vi "Main.vi"() -> ()   [LabVIEW 2020]
uses:
  Connection Info.ctl
  Command.ctl
  Shared/MySQL/Preset Query Enum.ctl
  <userlib>/_OpenG.lib/array/array.llb/Index 1D Array Elements (String)__ogtk.vi
  <vilib>/Utility/tcp.llb/UDP Multicast Write-Only Open.vi
panel:
  in  "clear list":bool
  in  "Multicolumn Listbox":i32[](listbox)
  out "x+y":dbl
  in  "MultiCast Port":u16=58432
  in  "Multicast Address":string="234.5.6.7"
  in  "Multicast Local Port":u16=58431
  in  "Who Alive":bool
  out "Devies To Stop":string[](array[string])
  out "NewVal":i32[](array[numeric])
  out "All connections":T1[](array[typedef])
  in  "SendStop":bool
  in  "Exit":bool
  in  "Listbox":i32[](listbox)
  in  "error in (no error)":errorcluster
  out "Variant Out 2":variant
  out "Received String":string
  out "after substring 2":string
  out "Entity Name":string
  out "Entity IP address":string
  out "before substring 2":string
  out "before substring":string
  out "after substring":string
  out "data out":string
  in  "port":u16=6341
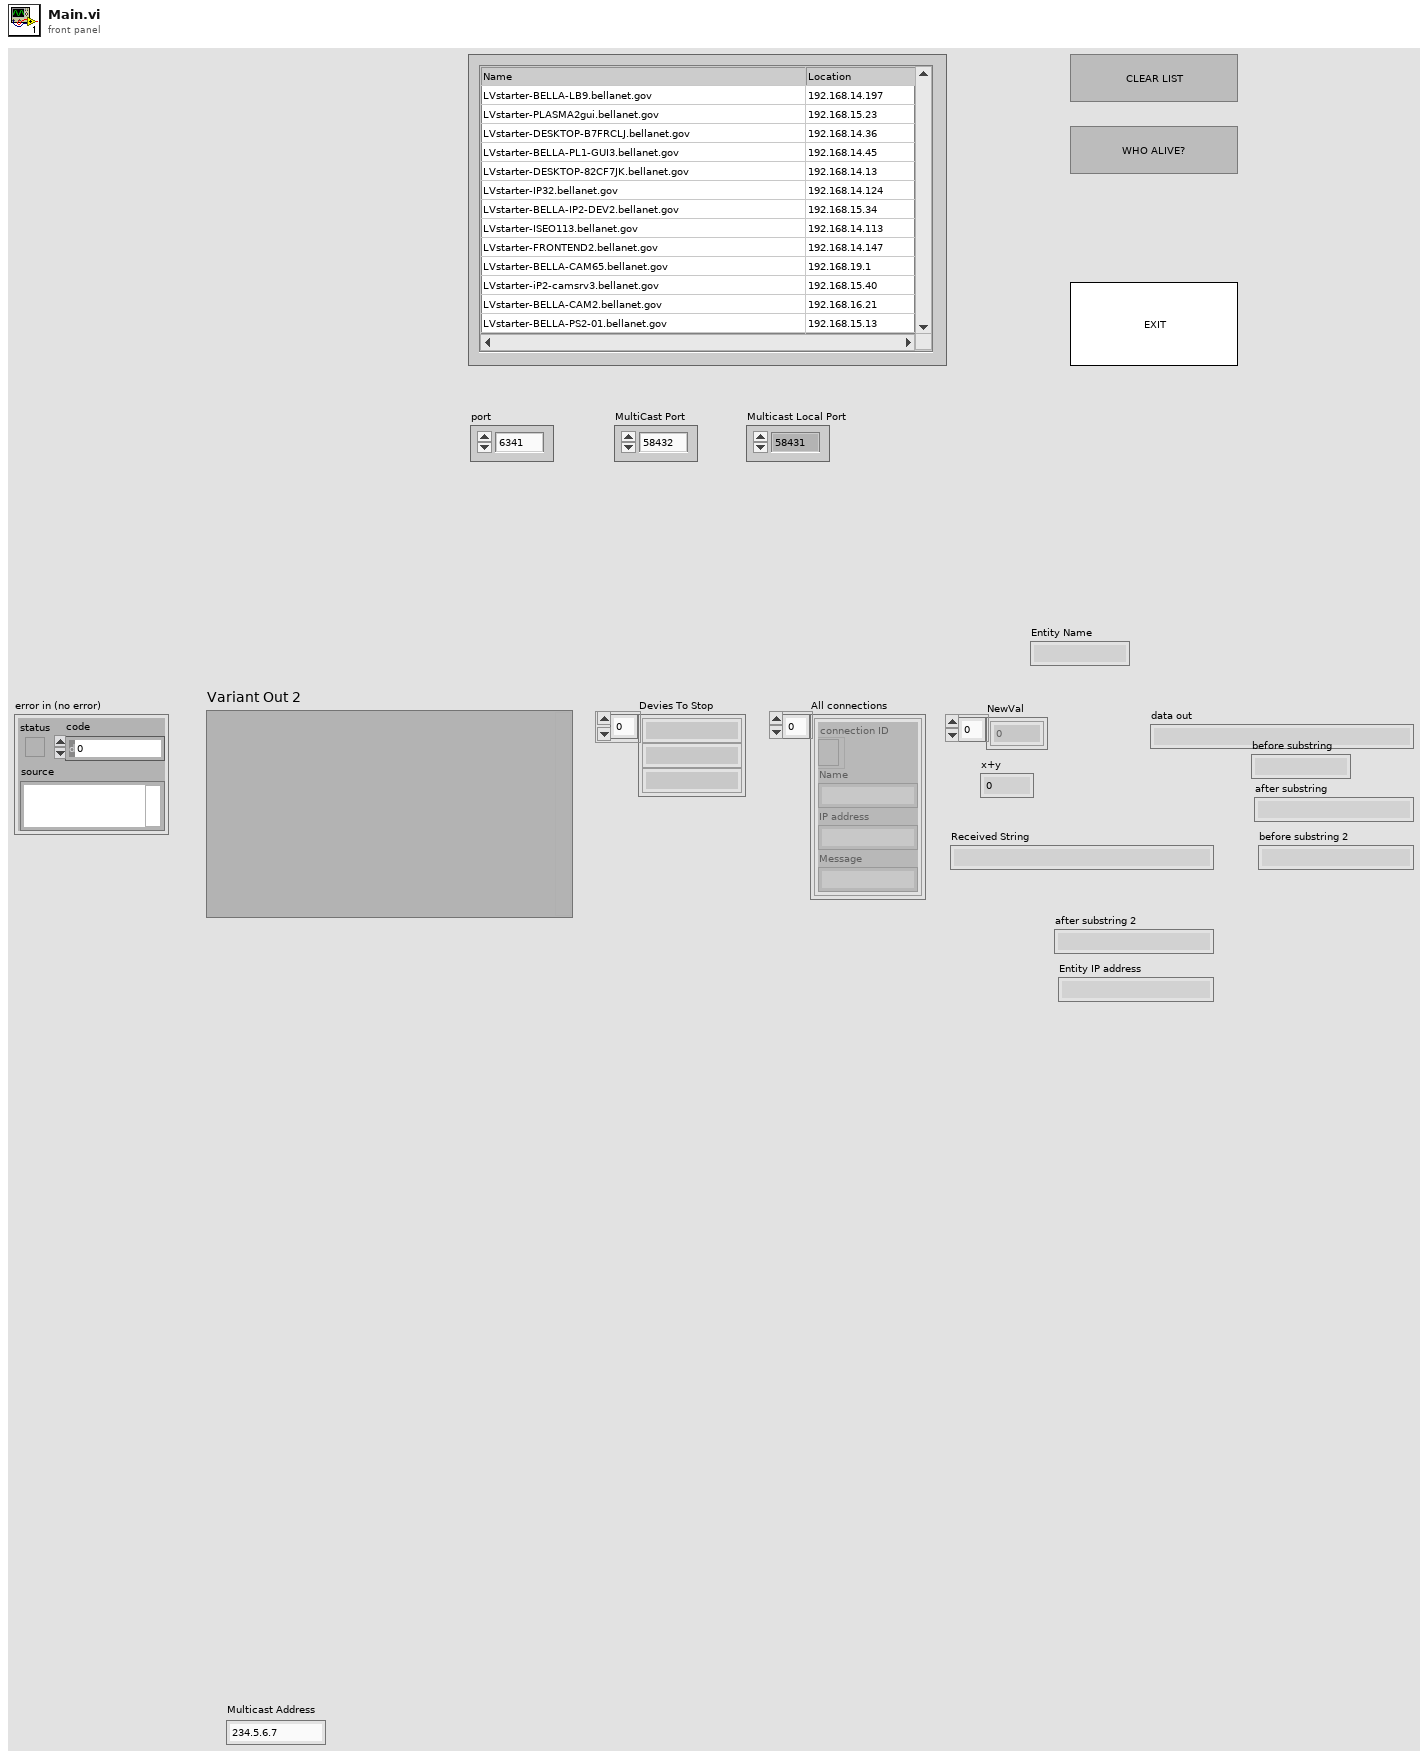
[diagram p1: front panel]
types:
  T1 = typedef "Connection Info.ctl" = cluster{"connection ID":refnum<k5>, "Name":string, "IP address":string, "Message":string}
  T2 = typedef "Command.ctl" = enum16{"add connection", "remove connection", "read connection data", "return all connections", "reset"}
  T3 = typedef "Preset Query Enum.ctl" = enum16{"Get Locations", "Get all IPs and MACs", "Get classes", "Get expt variables to set at scanstart for particular device", "Get expt devices and variables with start values", "Get expt devices and variables (with data to get)", "Get expt devices with data to get", "Get Expt devices and GUIs", "Get all devices basic properties", "Get Virtual Devices Core Info", "Get Expt names", "Get experiment basic properties", "Get experiment alarm variables", "Get MC Ports", "Get device network comm port", "Get devicetype lvclass path", "Get basic device properties", "Get Init Order", "Get all setable variables of a device", "Get device variable aliases", "Get force values of all settable variables", "Get all variables of a devicetype", "Get all variables of a device", "Get plotter details", "Get Saved Scans", "Get Scan Info", "GetGeneralGUIs", "Get expt for plotter", "Get plotter IDs from expt", "Get all devices", "Get all Virtual Devices", "Get all aliases", "Get variable and device info for Virtual Device", "GetItemLocatorIP", "Get IPs for GUIs", "Get DeviceType from Device", "GetLocalPortRange", "GetDevicePresetVariables", "Get Device Configuration", "GetAllPresetNames", "GetAllConfigurationNames", "GetPresetDeviceNames", "GetDeviceAliases", "GetDevicesOfClass"}
  T4 = enum32{"invalid app kind", "Development System", "Run Time System", "Student Edition", "Embedded LabVIEW", "Evaluation", "Custom"}
  T5 = enum32{"Invalid", "Standard", "Closed", "Hidden", "Minimized", "Maximized"}
  T6 = cluster{"Core":cluster{"Current VI Reference":refnum<vi>, "Close Panel on Exit?":bool}, "Your Boolean data":bool, "Your string data":string, "All connections":T1[], "Devies To Stop":string[], "MultiCast connection ID":refnum<k16>}
  T7 = cluster{"Current VI Reference":refnum<vi>, "Close Panel on Exit?":bool}
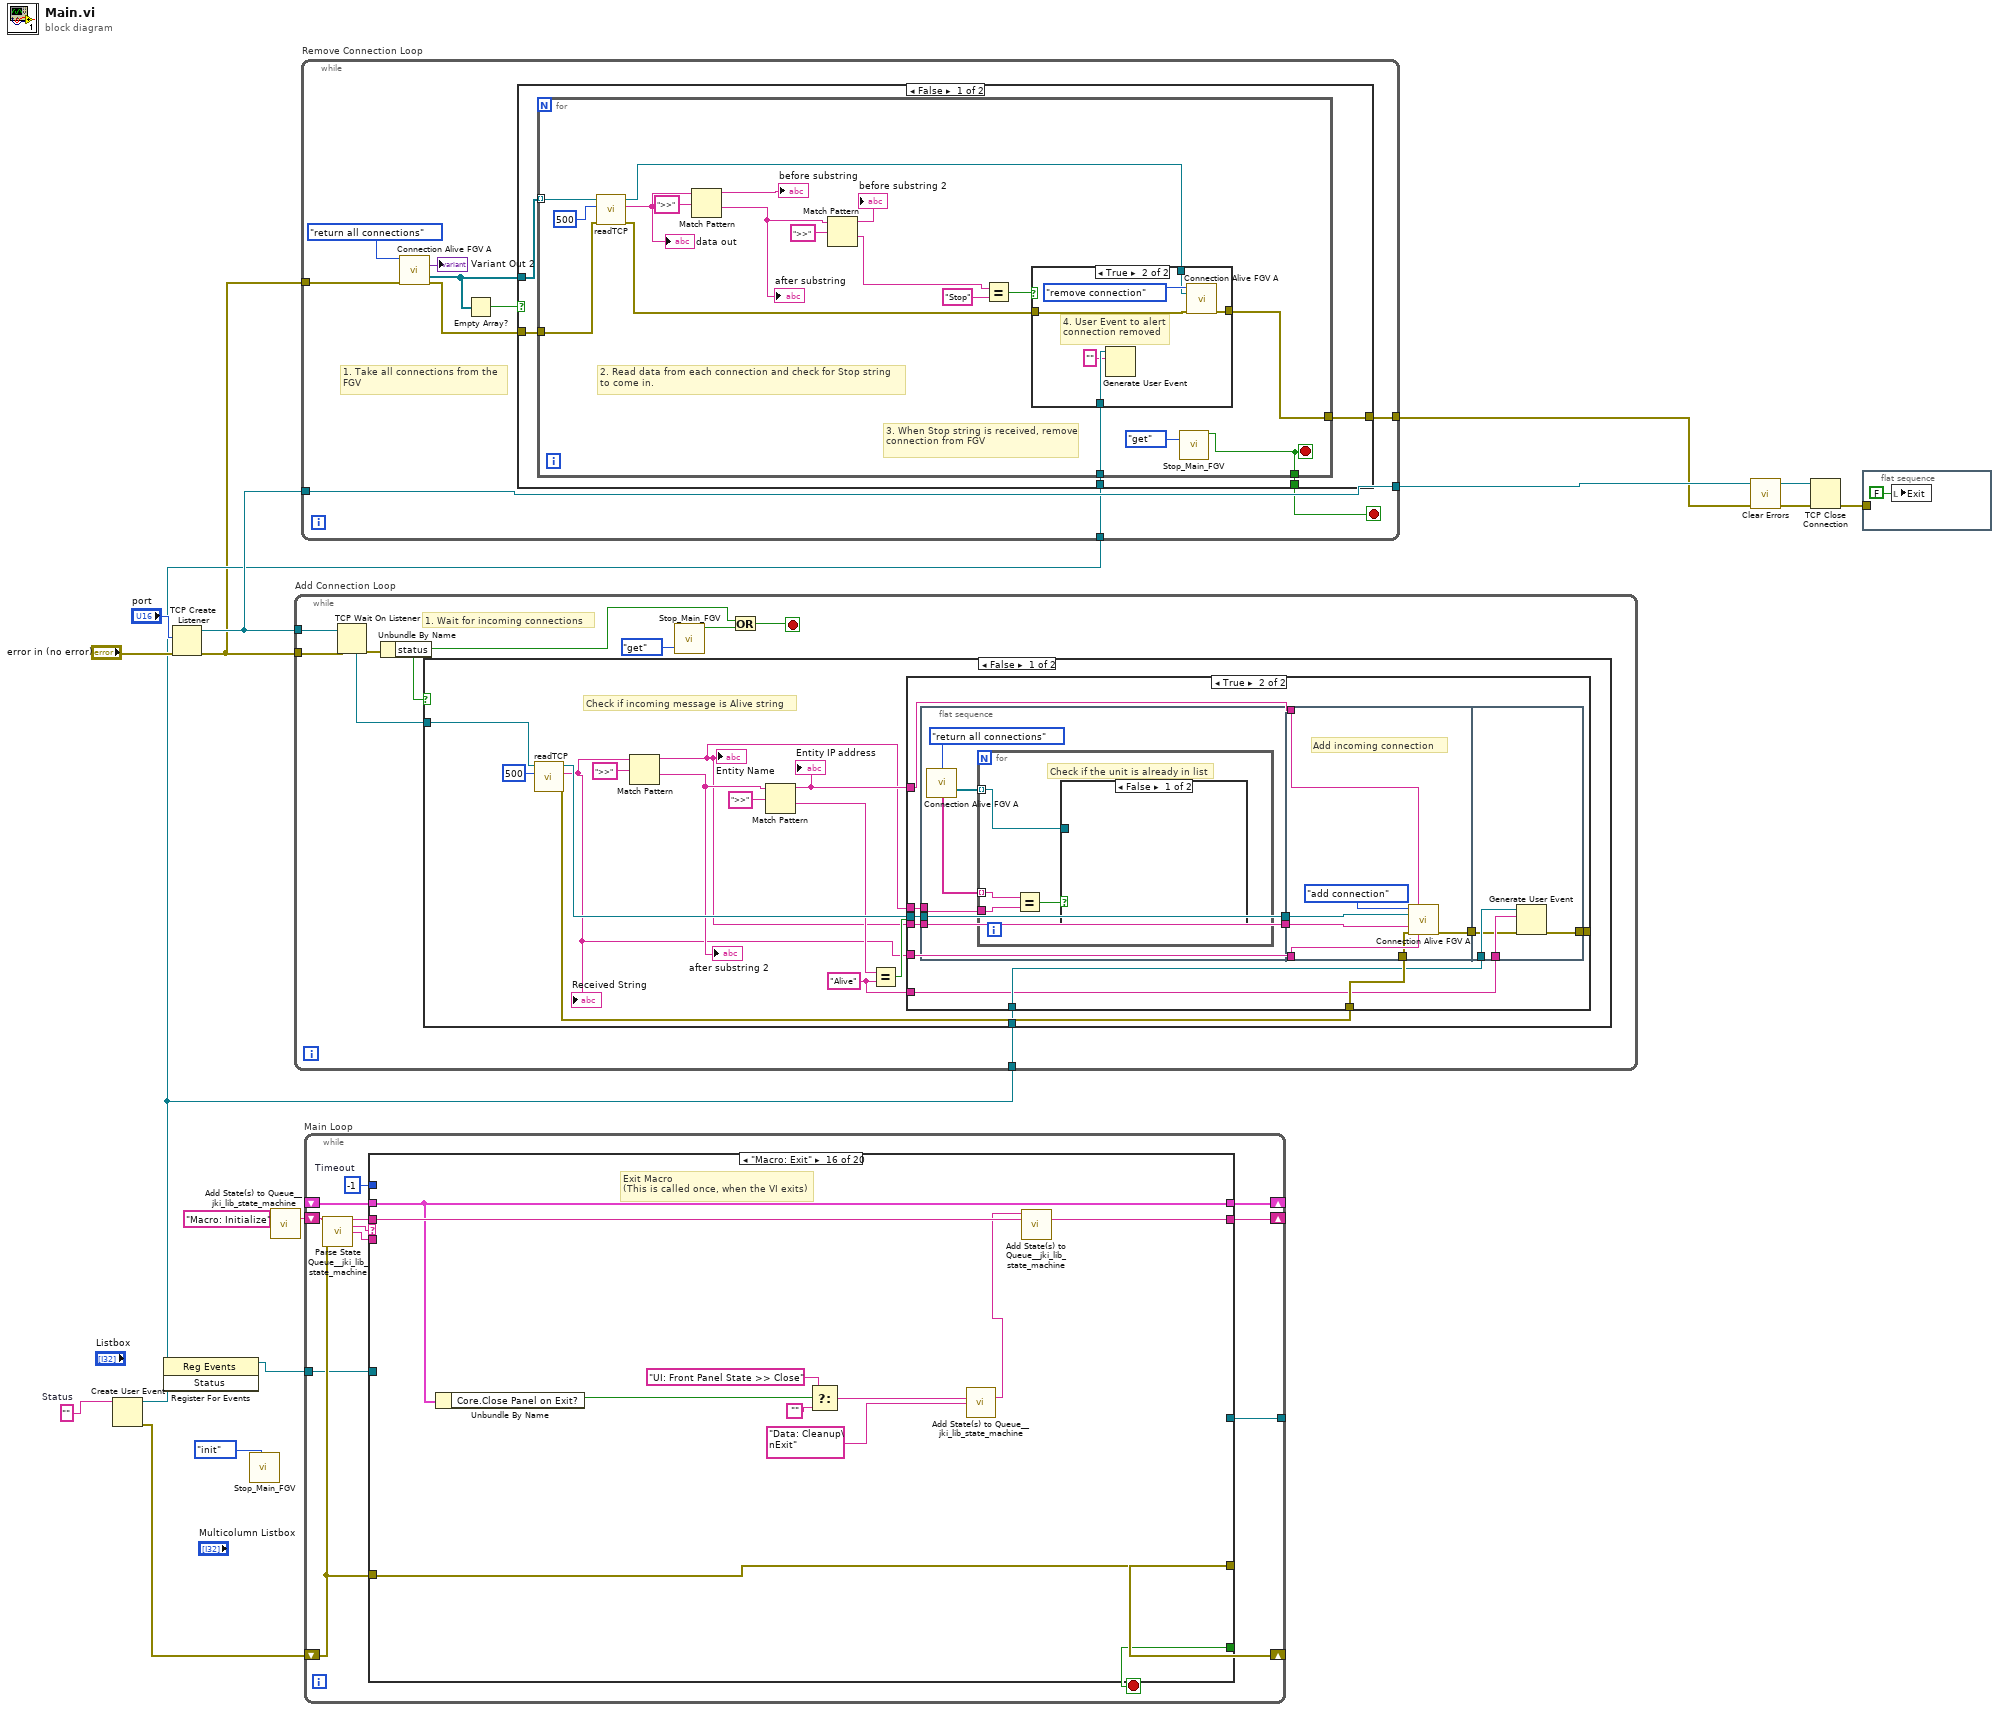
[diagram p0: block diagram]
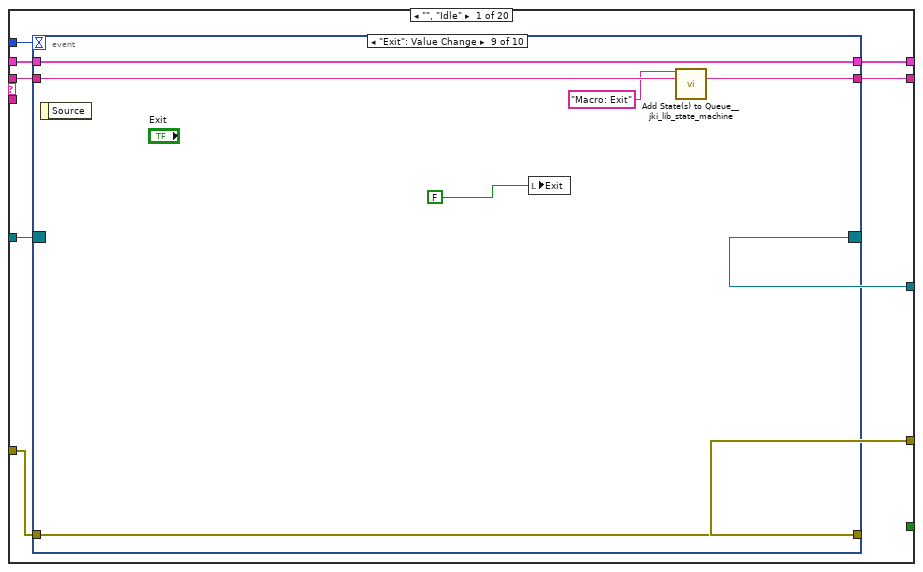
[diagram p2: hidden frame]
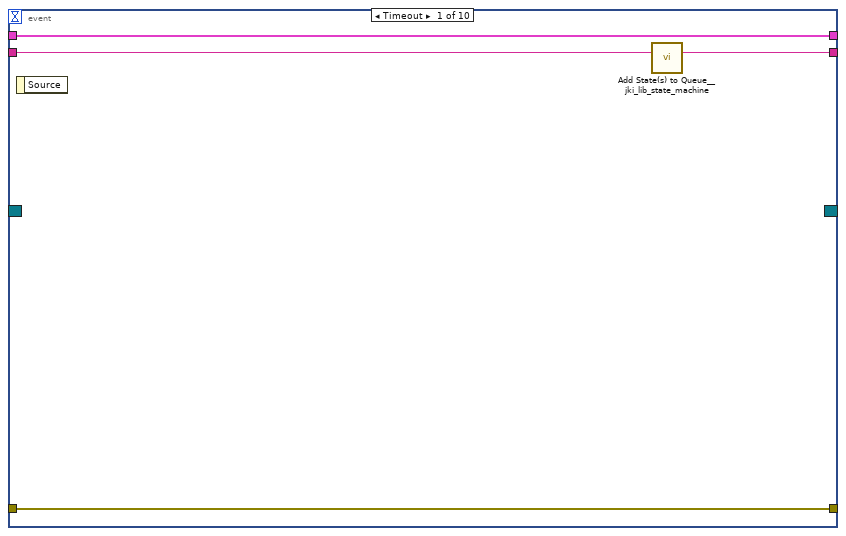
[diagram p3: hidden frame]
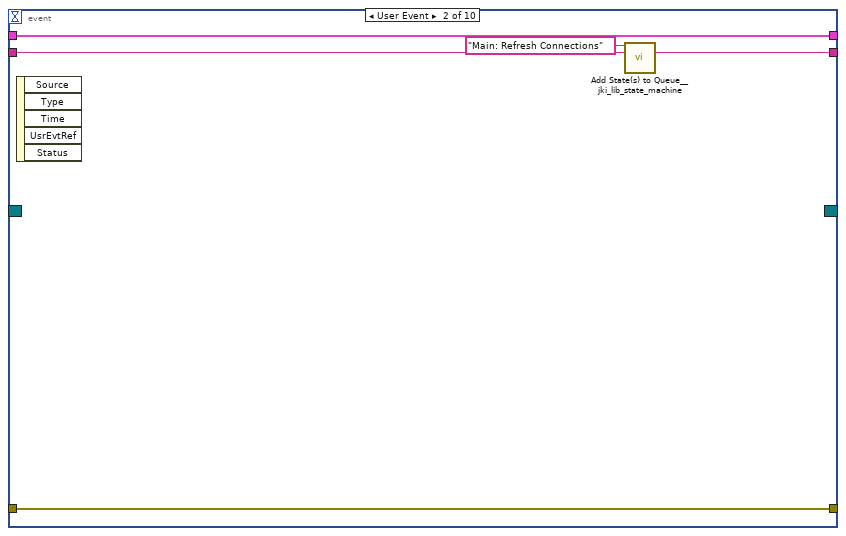
[diagram p4: hidden frame]
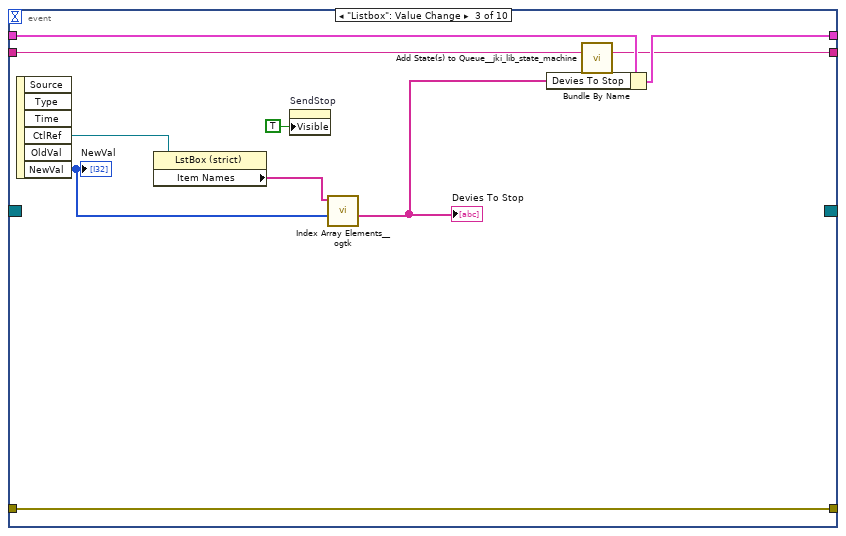
[diagram p5: hidden frame]
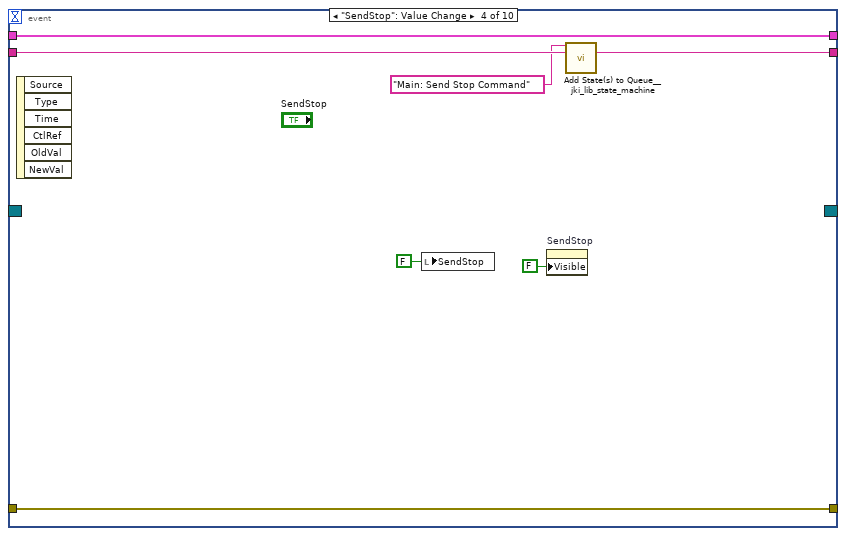
[diagram p6: hidden frame]
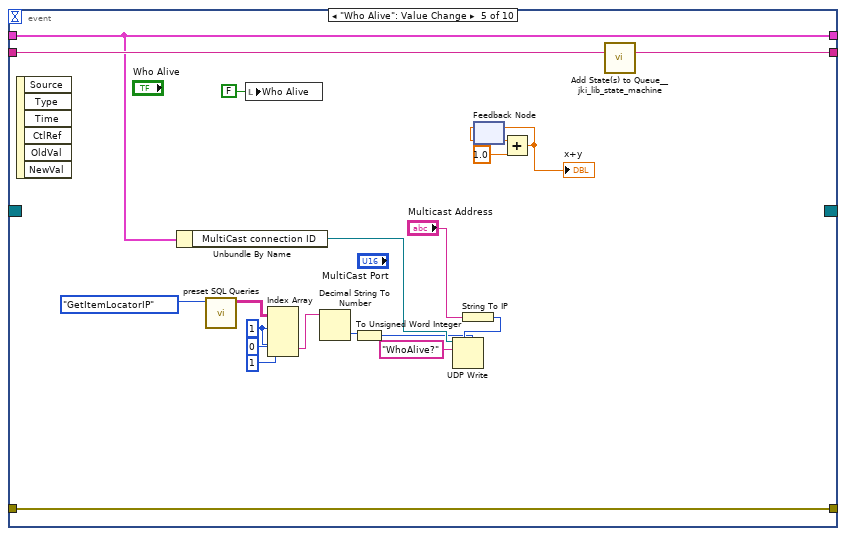
[diagram p7: hidden frame]
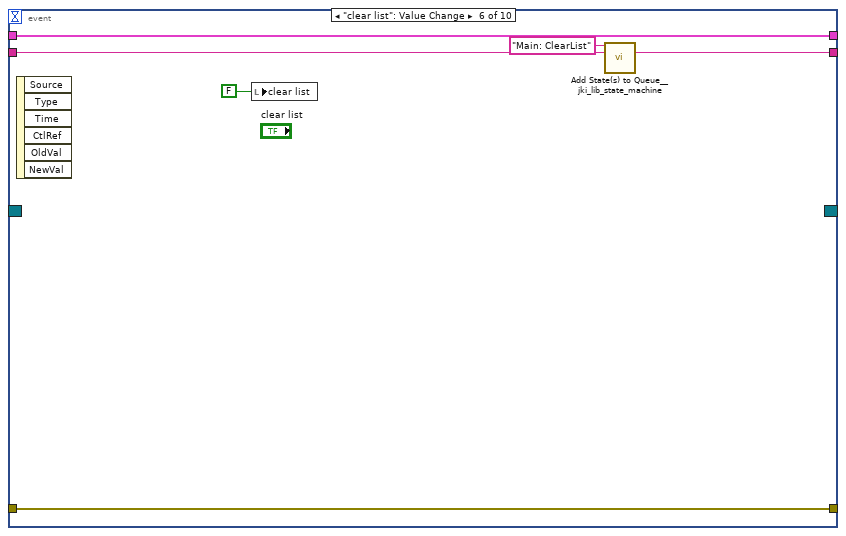
[diagram p8: hidden frame]
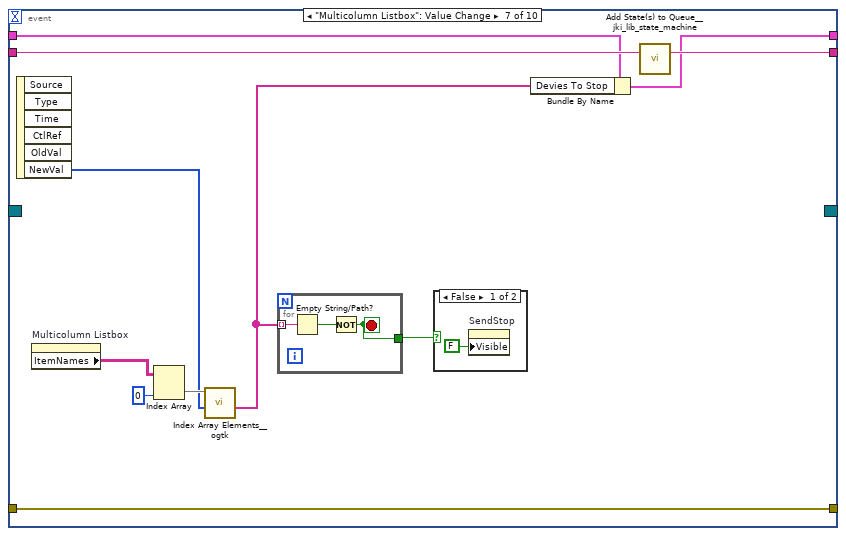
[diagram p9: hidden frame]
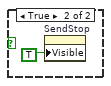
[diagram p10: hidden frame]
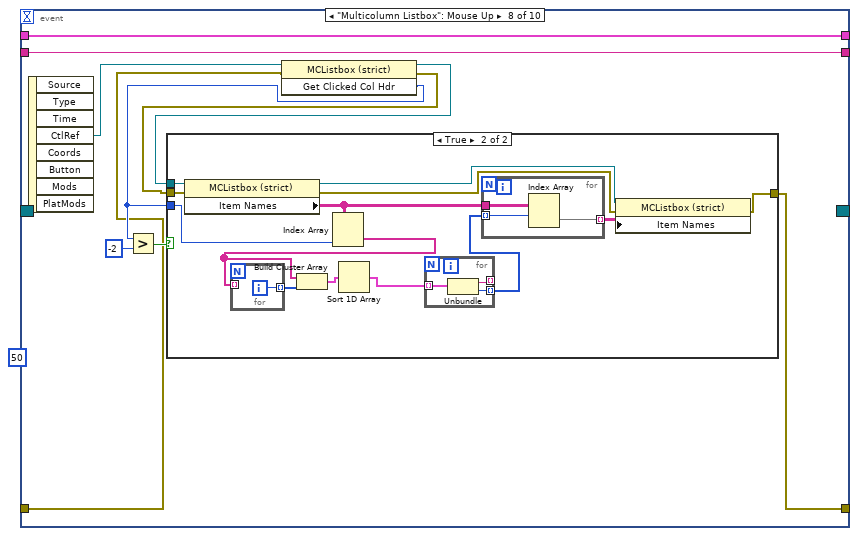
[diagram p11: hidden frame]
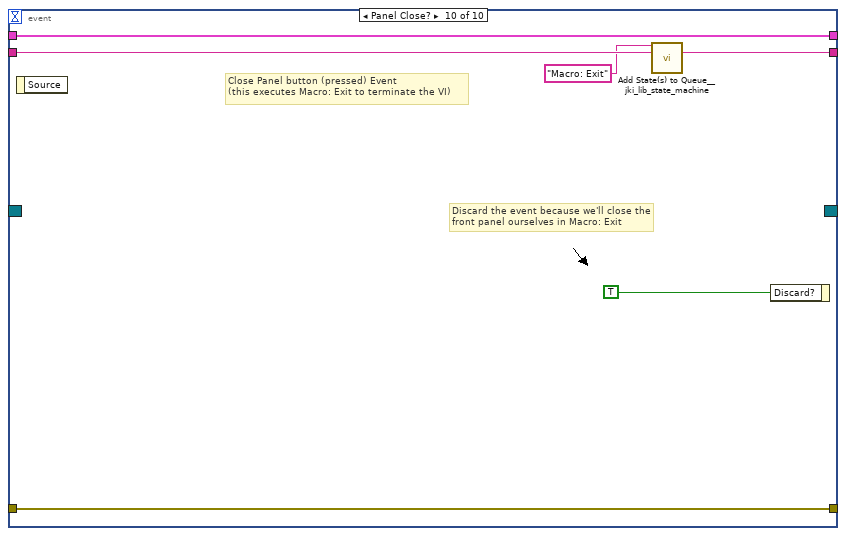
[diagram p13: hidden frame]
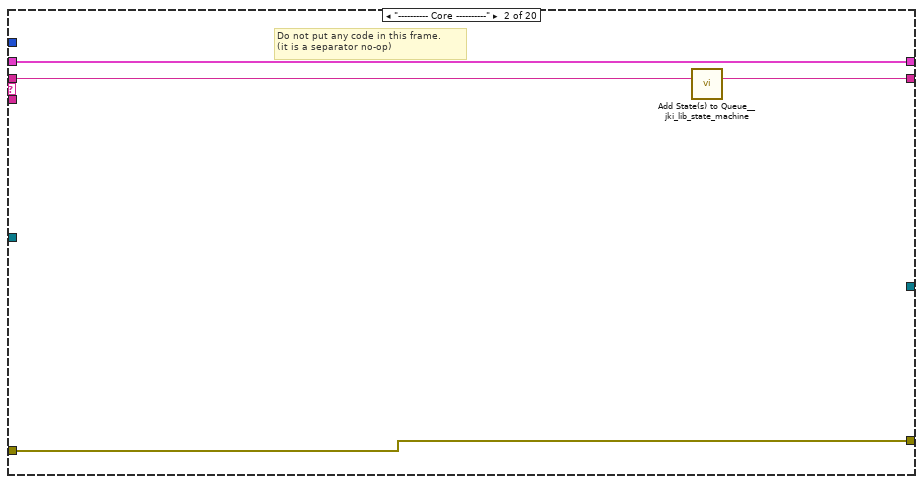
[diagram p14: hidden frame]
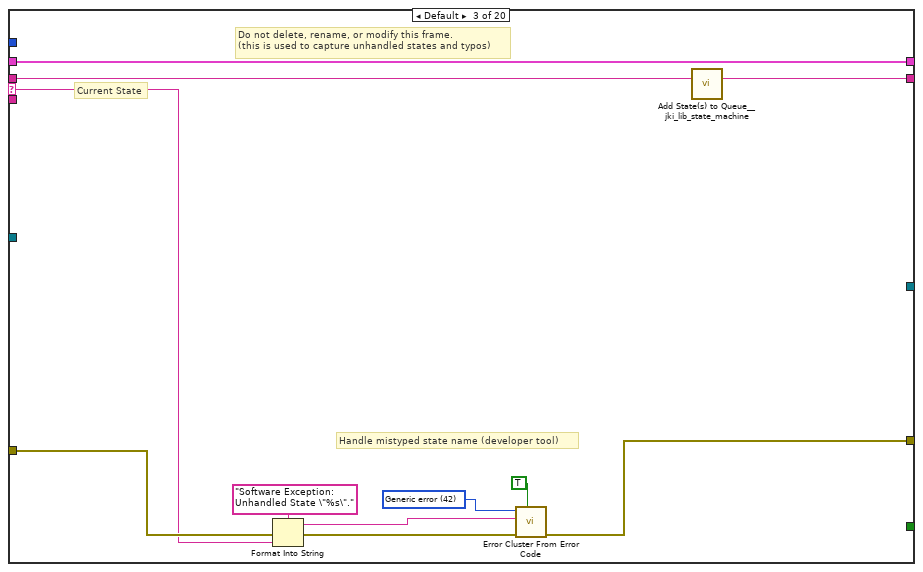
[diagram p15: hidden frame]
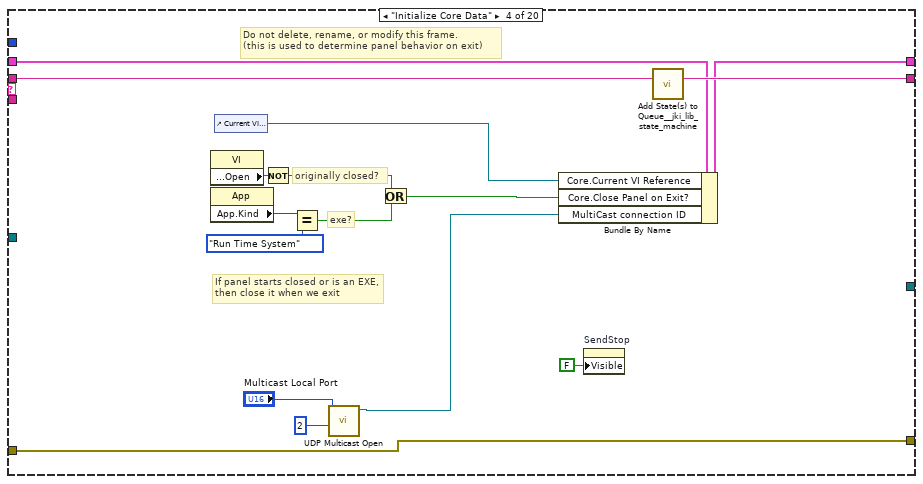
[diagram p16: hidden frame]
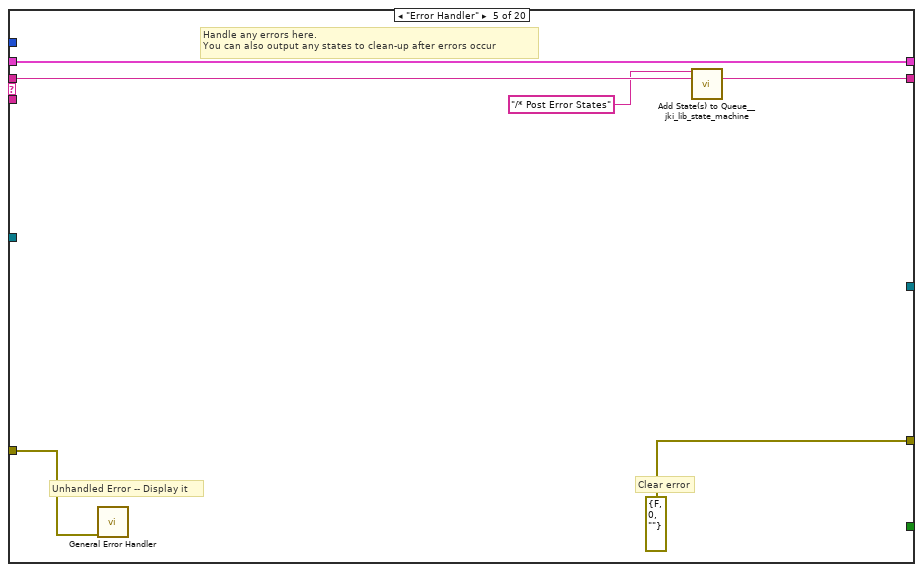
[diagram p17: hidden frame]
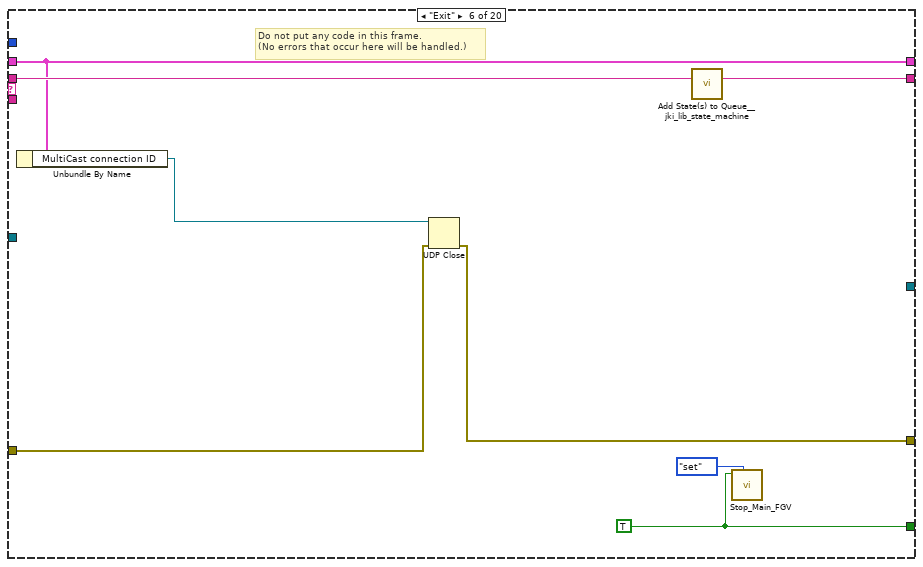
[diagram p18: hidden frame]
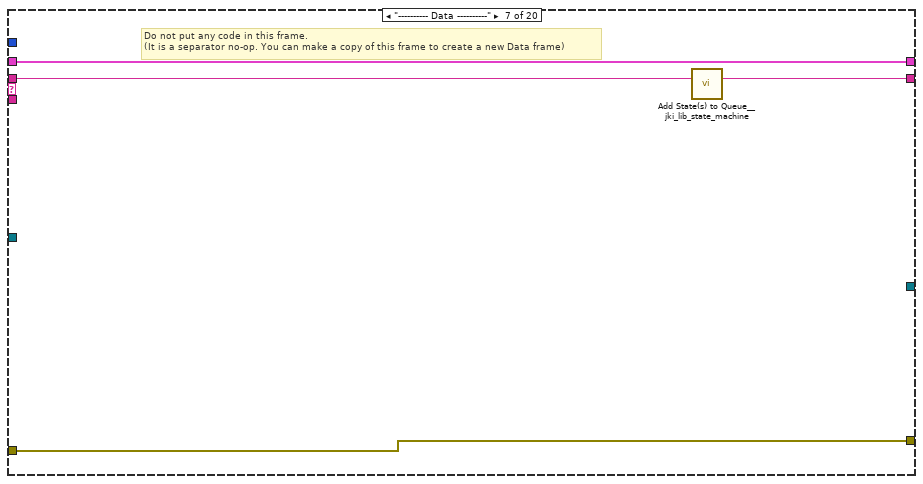
[diagram p19: hidden frame]
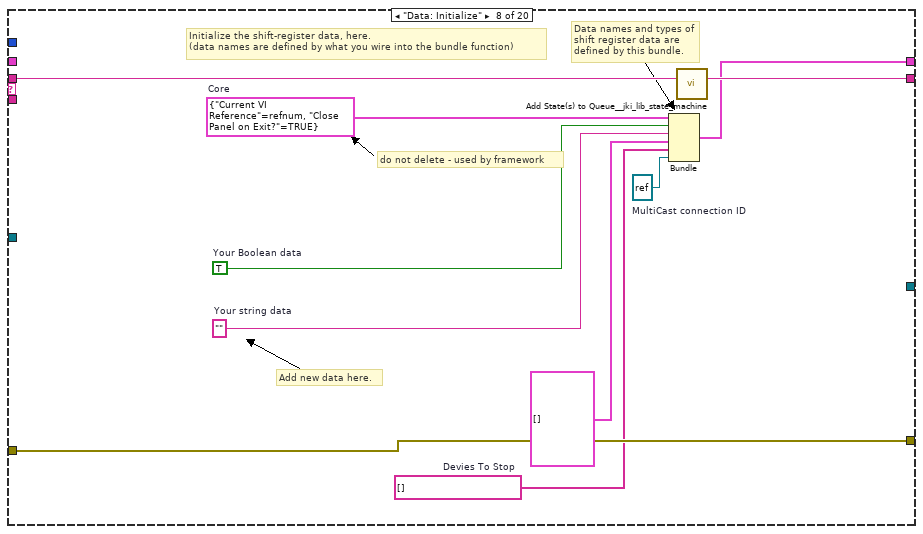
[diagram p20: hidden frame]
diagram:
  w6 = ""  # Status
  n1 = Create User Event(user event datatype=w6) -> (user event=w5:refnum<user-event>, error out=w3:errorcluster)  [unwired: 1 in]
  n2 = register-events(w5) -> (reference out=w7:refnum<event-registration>)  [unwired: 2 in, 1 out]
  n3 = TCP Create Listener(8:"error in (no error)", 10:"port") -> (0:w4:errorcluster, 3:w14:refnum<k5>)  [unwired: 4 out]
  n4 = call "Stop_Main_FGV.vi"("Command"=enum16{"set", "get", "init"}."init") -> ()  [unwired: 10 in, 1 out]
  n5 = call <vilib>:"Add State(s) to Queue__jki_lib_state_machine.vi"("State(s) in (\"\")"="Macro: Initialize") -> ("States Out"=w9:string)  [unwired: 14 in]
  n6 = while "Add Connection Loop" {
    tunnel: w4 -> [w24]
    tunnel: w14 -> [w23]
    tunnel: w5 -> [w20]
    stop <- w16 stop-if-true
    # "1. Wait for incoming connections"
    n7 = TCP Wait On Listener(8:w24, 11:w23) -> (0:w22:errorcluster, 4:w21:refnum<k5>)  [unwired: 5 out]
    n8 = Unbundle By Name(w22) -> ("status"=w17:bool)
    n9 = case shown="False" w17 {
      tunnel: w21 -> [w29 _]
      tunnel: w20 -> [w27 _]
      frame False {
        w26 = "Alive" ("y")
        # "Check if incoming message is Alive string"
        n10 = call "readTCP.vi"("timeout ms (-1)"=500, "connection ID in"=w29) -> ("error out"=w35:errorcluster, "data out"=w28:string, "connection ID out"=w37:refnum<k5>)  [unwired: 7 in]
        "Received String" <- w28
        n11 = Match Pattern(string=w28, regular expression=">>") -> (before substring=w25:string, after substring=w32:string)  [unwired: 1 in, 2 out]
        "after substring 2" <- w32
        "Entity Name" <- w25
        n12 = Match Pattern(string=w32, regular expression=">>") -> (before substring=w33:string, after substring=w36:string)  [unwired: 1 in, 2 out]
        "Entity IP address" <- w33
        n13 = Equal?(x=w36, y=w26) -> (x = y?=w34:bool)
        n14 = case shown="True" w34 {
          tunnel: w37 -> [_ w51]
          tunnel: w25 -> [_ w50]
          tunnel: w33 -> [_ w49]
          tunnel: [w39 w48] -> _
          tunnel: w28 -> [_ w47]
          tunnel: w35 -> [w39 w46]
          tunnel: w27 -> [_ w44]
          tunnel: w26 -> [_ w43]
          tunnel: w25 -> [_ w40]
          frame False {
          }
          frame True {
            n15 = flat-sequence {
              tunnel: w50 -> [w56]
              tunnel: w51 -> [w57]
              tunnel: [w57] -> w42
              tunnel: [w56] -> w41
              tunnel: w40 -> [w53]
              tunnel: w49 -> [w67]
              tunnel: w47 -> [w65]
              tunnel: w46 -> [w64]
              tunnel: [w66] -> w45
              tunnel: w42 -> [w70]
              tunnel: w41 -> [w68]
              tunnel: [w71] -> w48
              tunnel: w45 -> [w72]
              tunnel: w44 -> [w74]
              tunnel: w43 -> [w73]
              frame #0 {
                n16 = call "Connection Alive FGV A.vi"("command"=Command."return all connections") -> ("all connections"=w52:refnum<k5>[], "Names"=w54:string[])  [unwired: 7 in, 6 out]
                n17 = for {
                  tunnel: w54 -> [w61] mode=indexing
                  tunnel: w53 -> [w60]
                  tunnel: w52 -> [w58] mode=indexing
                  # "Check if the unit is already in list"
                  n18 = Equal?(x=w61, y=w60) -> (x = y?=w59:bool)
                  n19 = case shown="False" w59 {
                    tunnel: w58 -> [_ w62]
                    frame False {
                    }
                    frame True {
                      # "Remove existing connection"
                      n20 = call "Connection Alive FGV A.vi"("command"=Command."remove connection", "connection ID"=w62) -> ()  [unwired: 6 in, 8 out]
                    }
                  }
                }
              }
              frame #1 {
                # "Add incoming connection"
                n21 = call "Connection Alive FGV A.vi"("command"=Command."add connection", "IP address"=w67, "connection ID"=w70, "Name"=w68, "error in (no error)"=w64, "Message"=w65) -> ("error out"=w66:errorcluster)  [unwired: 2 in, 7 out]
              }
              frame #2 {
                n22 = Generate User Event(user event=w74, event data cluster=w73, error in=w72) -> (error out=w71:errorcluster)  [unwired: 1 in, 1 out]
              }
            }
          }
        }
      }
      frame True {
      }
    }
    n23 = call "Stop_Main_FGV.vi"("Command"=enum16{"set", "get", "init"}."get") -> ("Stop out"=w18:bool)  [unwired: 10 in]
    n24 = Or(x=w17, y=w18) -> (x .or. y?=w16:bool)
  }
  n25 = while "Remove Connection Loop" {
    tunnel: w14 -> [w80]
    tunnel: [w80] -> w13
    tunnel: [w79] -> w12
    tunnel: w5 -> [w77]
    tunnel: w4 -> [w76]
    stop <- w75 stop-if-true
    # "1. Take all connections from the \nFGV"
    n26 = call "Connection Alive FGV A.vi"("command"=Command."return all connections", "error in (no error)"=w76) -> ("Variant Out"=→"Variant Out 2":variant, "all connections"=w82:refnum<k5>[], "error out"=w83:errorcluster)  [unwired: 6 in, 5 out]
    n27 = Empty Array?(array=w82) -> (empty?=w81:bool)
    n28 = case shown="False" w81 {
      tunnel: w83 -> [w89 w117]
      tunnel: w82 -> [w88 _]
      tunnel: [w87 w117] -> w79
      tunnel: w77 -> [w86 _]
      tunnel: [w85 w115] -> w75
      frame False {
        n29 = for {
          tunnel: w88 -> [w107] mode=indexing
          tunnel: w89 -> [w96]
          tunnel: [w94] -> w87
          tunnel: w86 -> [w92]
          tunnel: [w90] -> w85
          stop <- w90 stop-if-true
          # "3. When Stop string is received, remove connection from FGV"
          # "2. Read data from each connection and check for Stop string\nto come in."
          n30 = call "readTCP.vi"("error in (no error)"=w96, "timeout ms (-1)"=500, "connection ID in"=w107) -> ("error out"=w95:errorcluster, "data out"=w93:string, "connection ID out"=w98:refnum<k5>)  [unwired: 6 in]
          "data out" <- w93
          n31 = Match Pattern(string=w93, regular expression=">>") -> (before substring=→"before substring":string, after substring=w103:string)  [unwired: 1 in, 2 out]
          "after substring" <- w103
          n32 = Match Pattern(string=w103, regular expression=">>") -> (before substring=→"before substring 2":string, after substring=w100:string)  [unwired: 1 in, 2 out]
          n33 = Equal?(x=w100, y="Stop") -> (x = y?=w99:bool)
          n34 = case shown="True" w99 {
            tunnel: w98 -> [_ w113]
            tunnel: [w108 w112] -> w94
            tunnel: w95 -> [w108 w111]
            tunnel: w92 -> [_ w110]
            frame False {
            }
            frame True {
              # "4. User Event to alert\nconnection removed"
              n35 = Generate User Event(user event=w110, event data cluster="" ("event data")) -> ()  [unwired: 2 in, 2 out]
              n36 = call "Connection Alive FGV A.vi"("command"=Command."remove connection", "connection ID"=w113, "error in (no error)"=w111) -> ("error out"=w112:errorcluster)  [unwired: 5 in, 7 out]
            }
          }
          n37 = call "Stop_Main_FGV.vi"("Command"=enum16{"set", "get", "init"}."get") -> ("Stop out"=w90:bool)  [unwired: 10 in]
        }
      }
      frame True {
        n38 = call "Stop_Main_FGV.vi"("Command"=enum16{"set", "get", "init"}."get") -> ("Stop out"=w115:bool)  [unwired: 10 in]
      }
    }
  }
  n39 = while "Main Loop" {
    shift-right: [w123] -> _
    shift-left: _ -> [w122]
    shift-right: [w126] -> _
    shift-left: w3 -> [w120]
    shift-right: [w125] -> _
    shift-left: w9 -> [w127]
    tunnel: w7 -> [w119]
    tunnel: [w118] -> _
    stop <- w124 stop-if-true
    w121 = -1  # Timeout
    n40 = call <vilib>:"Parse State Queue__jki_lib_state_machine.vi"("State Queue"=w127, "Error In (no error)"=w120) -> ("Remaining States"=w129:string, "Current State"=w130:string, "Arguments"=w128:string)  [unwired: 11 in]
    n41 = case shown="\"Macro: Exit\"" w130 {
      selector: w130 -> [_ _ w255 _ _ _ _ _ _ _ _ _ _ _ _ _ _ _ _ _]
      tunnel: w129 -> [w139 w254 w259 w281 w287 w295 w299 w309 w315 w319 w323 w329 w340 w366 w371 w381 w385 w391 w417 w432]
      tunnel: w128 -> [_ _ _ _ _ _ _ _ _ _ _ w324 w334 _ _ _ _ _ _ _]
      tunnel: w122 -> [w137 w251 w257 w272 w284 w293 w296 _ w310 w316 w321 w327 w336 w363 w368 w378 w382 w388 w414 w421]
      tunnel: [w136 w252 w261 w278 errorcluster {"status"=FALSE, "code"=0, "source"=""} ("error out") w290 w297 w306 w311 w317 w320 w325 w337 w364 w369 w379 w383 w389 w415 w430] -> w126
      tunnel: w120 -> [w135 w252 w260 w278 w283 w291 w297 w306 w312 w317 w320 w326 w338 w364 w369 w379 w383 w389 w415 w430]
      tunnel: [w138 w253 w258 w280 w286 w294 w298 w308 w314 w318 w322 w328 w339 w365 w370 w380 w384 w390 w416 w431] -> w125
      tunnel: [_ _ _ _ _ w289 _ _ _ _ _ _ _ _ _ _ _ _ _ _] -> w124
      tunnel: [w134 w251 w257 w279 w284 w293 w296 w307 w310 w316 w321 w327 w336 w363 w368 w378 w382 w388 w414 w420] -> w123
      tunnel: w121 -> [w133 _ _ _ _ _ _ _ _ _ _ _ _ _ _ _ _ _ _ _]
      tunnel: w119 -> [w132 _ _ _ _ _ _ _ _ _ _ _ _ _ _ _ _ _ _ _]
      tunnel: [w131 _ _ _ _ _ _ _ _ _ _ _ _ _ _ _ _ _ _ _] -> w118
      frame "", "Idle" {
        n42 = event shown="[8] \"Exit\": Value Change" {
          selector: w132 -> [_ _ _ _ _ _ _ _ _ _]
          dyn-events: [_ _ _ _ _ _ _ _ _ _] -> w131
          timeout: w133 -> [_ _ _ _ _ _ _ _ _ _]
          tunnel: w139 -> [w143 w146 w150 w163 w179 w188 w201 w208 w244 w250]
          tunnel: [w142 w147 w149 w162 w180 w189 w202 w208 w243 w249] -> w138
          tunnel: w137 -> [w140 w144 w153 w165 w178 w187 w195 w209 w241 w247]
          tunnel: [w141 w148 w157 w164 w181 w190 w198 w210 w242 w248] -> w136
          tunnel: w135 -> [w141 w148 w157 w164 w181 w190 w198 w213 w242 w248]
          tunnel: [w140 w144 w152 w165 w178 w187 w194 w209 w241 w247] -> w134
          event Timeout {
            n43 = event-data() -> ()  [unwired: 1 in, 1 out]
            n44 = call <vilib>:"Add State(s) to Queue__jki_lib_state_machine.vi"("State(s) in (\"\")"=w143) -> ("States Out"=w142:string)  [unwired: 14 in]
          }
          event User Event {
            n45 = event-data() -> ()  [unwired: 1 in, 5 out]
            n46 = call <vilib>:"Add State(s) to Queue__jki_lib_state_machine.vi"("State(s) in Front (\"\")"="Main: Refresh Connections" ("State(s) in Front (\"\")"), "State(s) in (\"\")"=w146) -> ("States Out"=w147:string)  [unwired: 13 in]
          }
          event "Listbox": Value Change {
            n47 = event-data() -> ("CtlRef"=w156:refnum<vi>, "NewVal"=w154:i32[])  [unwired: 1 in, 4 out]
            "NewVal" <- w154
            n48 = property class="LstBox (strict)"(reference=w156) -> ("Item Names"=w155:string[])  [unwired: 1 in, 2 out]
            n49 = property on="SendStop" class="Bool (strict)"("Visible"=TRUE) -> ()  [unwired: 2 in, 2 out]
            n50 = call-poly <userlib>:"Index Array Elements__ogtk.vi"("indices"=w154, "array"=w155) -> ("elements"=w151:string[])  [unwired: 9 in]
            "Devies To Stop" <- w151
            n51 = Bundle By Name(cluster=w153, "Devies To Stop"=w151) -> (w152:T6)
            n52 = call <vilib>:"Add State(s) to Queue__jki_lib_state_machine.vi"("State(s) in (\"\")"=w150) -> ("States Out"=w149:string)  [unwired: 14 in]
          }
          event "SendStop": Value Change {
            n53 = event-data() -> ()  [unwired: 1 in, 6 out]
            n54 = local write "SendStop"(FALSE ("OK 2")) -> ()
            n55 = property on="SendStop" class="Bool (strict)"("Visible"=FALSE) -> ()  [unwired: 2 in, 2 out]
            n56 = call <vilib>:"Add State(s) to Queue__jki_lib_state_machine.vi"("State(s) in Front (\"\")"="Main: Send Stop Command" ("State(s) in Front (\"\")"), "State(s) in (\"\")"=w163) -> ("States Out"=w162:string)  [unwired: 13 in]
          }
          event "Who Alive": Value Change {
            w168 = 1 ("index (row)")
            n57 = event-data() -> ()  [unwired: 1 in, 6 out]
            n58 = Unbundle By Name(w178) -> ("MultiCast connection ID"=w177:refnum<k16>)
            n59 = call "preset SQL Queries.vi"("Preset Query"=Preset_Query_Enum."GetItemLocatorIP") -> ("data"=w167:string[][])  [unwired: 8 in, 2 out]
            n60 = local write "Who Alive"(FALSE ("Who Alive")) -> ()
            n61 = Index Array(array=w167, index (row) #1=w168, index (col) #1=0 ("disabled index (col)"), index (row) #2=w168, index (col) #2=1 ("disabled index (col)")) -> (element #2=w166:string)  [unwired: 1 out]
            n62 = Decimal String To Number(string=w166) -> (number=w172:i32)  [unwired: 2 in, 1 out]
            n63 = To Unsigned Word Integer(number=w172) -> (unsigned 16bit integer=w171:u16)
            n64 = String To IP(1:"Multicast Address") -> (0:w183:u32)
            n65 = UDP Write(address=w183, port or service name=w171, connection ID=w177, data in="WhoAlive?") -> ()  [unwired: 2 in, 2 out]
            n66 = feedback #1() -> (w175:dbl)  [unwired: 1 in]
            n67 = Add(x=w175, y=1.0) -> (x+y=w176:dbl)
            "x+y" <- w176
            n68 = feedback-in #1(w176) -> ()
            n69 = call <vilib>:"Add State(s) to Queue__jki_lib_state_machine.vi"("State(s) in (\"\")"=w179) -> ("States Out"=w180:string)  [unwired: 14 in]
          }
          event "clear list": Value Change {
            n70 = event-data() -> ()  [unwired: 1 in, 6 out]
            n71 = local write "clear list"(FALSE ("Who Alive")) -> ()
            n72 = call <vilib>:"Add State(s) to Queue__jki_lib_state_machine.vi"("State(s) in Front (\"\")"="Main: ClearList" ("State(s) in Front (\"\")"), "State(s) in (\"\")"=w188) -> ("States Out"=w189:string)  [unwired: 13 in]
          }
          event "Multicolumn Listbox": Value Change {
            n73 = event-data() -> ("NewVal"=w196:i32[])  [unwired: 1 in, 5 out]
            n74 = property on="Multicolumn Listbox" class="MCListbox (strict)"() -> ("ItemNames"=w200:string[][])  [unwired: 2 in, 2 out]
            n75 = Index Array(array=w200, index (col)=0 ("disabled index (col)")) -> (element=w197:string[])  [unwired: 1 in]
            n76 = call-poly <userlib>:"Index Array Elements__ogtk.vi"("indices"=w196, "array"=w197) -> ("elements"=w193:string[])  [unwired: 9 in]
            n77 = for {
              tunnel: w193 -> [w207] mode=indexing
              tunnel: [w205] -> w192
              stop <- w205 stop-if-true
              n78 = Empty String/Path?(string/path=w207) -> (empty?=w206:bool)
              n79 = Not(x=w206) -> (.not. x?=w205:bool)
            }
            n80 = case shown="False" w192 {
              frame False {
                n81 = property on="SendStop" class="Bool (strict)"("Visible"=FALSE) -> ()  [unwired: 2 in, 2 out]
              }
              frame True {
                n82 = property on="SendStop" class="Bool (strict)"("Visible"=TRUE) -> ()  [unwired: 2 in, 2 out]
              }
            }
            n83 = Bundle By Name(cluster=w195, "Devies To Stop"=w193) -> (w194:T6)
            n84 = call <vilib>:"Add State(s) to Queue__jki_lib_state_machine.vi"("State(s) in (\"\")"=w201) -> ("States Out"=w202:string)  [unwired: 14 in]
          }
          event "Multicolumn Listbox": Mouse Up {
            (unwired) u32 50 ("milliseconds to wait")
            n85 = event-data() -> ("CtlRef"=w215:refnum<vi>)  [unwired: 1 in, 7 out]
            n86 = invoke class="MCListbox (strict)" method="Get Clicked Col Hdr"(reference=w215, error in=w213) -> (reference out=w212:refnum<vi>, error out=w211:errorcluster, "Get Clicked Column Header"=w214:i32)  [unwired: 1 in]
            n87 = Greater?(x=w214, y=-2) -> (0:w217:bool)
            n88 = case shown="True" w217 {
              tunnel: w214 -> [_ w231]
              tunnel: w211 -> [w218 w224]
              tunnel: w212 -> [_ w230]
              tunnel: [w218 w225] -> w210
              frame False {
              }
              frame True {
                n89 = property class="MCListbox (strict)"(reference=w230, error in=w224) -> (reference out=w226:refnum<vi>, error out=w227:errorcluster, "Item Names"=w229:string[][])
                n90 = Index Array(array=w229, index (col)=w231) -> (element=w220:string[])  [unwired: 1 in]
                n91 = for {
                  tunnel: [w235] -> w221 mode=indexing
                  tunnel: w220 -> [_] mode=indexing
                  i -> [w235]
                }
                n92 = Build Cluster Array ("Index & Bundle Cluster Array")(w220, w221) -> (w222:cluster{string, i32}[])
                n93 = Sort 1D Array(array=w222) -> (sorted array=w223:cluster{string, i32}[])
                n94 = for {
                  tunnel: w223 -> [w234] mode=indexing
                  tunnel: [w233] -> _ mode=indexing
                  tunnel: [w232] -> w219 mode=indexing
                  n95 = Unbundle(w234) -> (w233:string, w232:i32)
                }
                n96 = for {
                  tunnel: w219 -> [w237] mode=indexing
                  tunnel: w229 -> [w238]
                  tunnel: [w236] -> w228 mode=indexing
                  n97 = Index Array(array=w238, index (row)=w237) -> (element=w236:string[])  [unwired: 1 in]
                }
                n98 = property class="MCListbox (strict)"(reference=w226, error in=w227, "Item Names"=w228) -> (error out=w225:errorcluster)  [unwired: 1 out]
              }
            }
          }
          event "Exit": Value Change {
            n99 = event-data() -> ()  [unwired: 1 in, 1 out]
            n100 = local write "Exit"(FALSE ("OK")) -> ()
            n101 = call <vilib>:"Add State(s) to Queue__jki_lib_state_machine.vi"("State(s) in Front (\"\")"="Macro: Exit", "State(s) in (\"\")"=w244) -> ("States Out"=w243:string)  [unwired: 13 in]
          }
          event Panel Close? {
            # "Discard the event because we'll close the front panel ourselves in Macro: Exit"
            # "Close Panel button (pressed) Event\n(this executes Macro: Exit to terminate the VI)"
            n102 = event-data() -> ()  [unwired: 1 in, 1 out]
            n103 = call <vilib>:"Add State(s) to Queue__jki_lib_state_machine.vi"("State(s) in Front (\"\")"="Macro: Exit", "State(s) in (\"\")"=w250) -> ("States Out"=w249:string)  [unwired: 13 in]
            n104 = event-data("Discard?"=TRUE) -> ()  [unwired: 1 in, 1 out]
          }
        }
      }
      frame "---------- Core ----------" {
        # "Do not put any code in this frame.\n(it is a separator no-op)"
        n105 = call <vilib>:"Add State(s) to Queue__jki_lib_state_machine.vi"("State(s) in (\"\")"=w254) -> ("States Out"=w253:string)  [unwired: 14 in]
      }
      frame Default {
        w264 = 42 items=["No error", "Argument error", "Memory is full", "Out of zone", "End of file", "File already open", "Generic file I/O error", "File not found", "File permission error", "Disk is full", "Duplicate path", "Too many files open", "System feature not enabled", "Resource file not found", "Cannot add resource", "Resource not found", "Image not found", "Image memory error", "Pen does not exist", "Config type invalid", "Config token not found", "Config parse error", "Config memory error", "Bad external code format", "Bad external code offset", "External code not present", "Null window", "Destroy window error", "Null menu", "Print aborted", "Bad print record", "Print driver error", "Windows error during printing", "Memory error during printing", "Print dialog error", "Generic print error", "Invalid device refnum", "Device not found", "Device parameter error", "Device unit error", "Cannot open device", "Device call aborted", "Generic error", "Cancelled by user", "Object ID too low", "Object ID too high", "Object not in heap", "Unknown heap", "Unknown object (invalid DefProc)", "Unknown object (DefProc not in table)", "Message out of range", "Invalid (null) method", "Unknown message", "Manager call not supported", "Bad address", "Network operation in progress", "Network operation timed out", "Connection is busy", "Network attribute not supported", "Network error", "Address in use", "System out of memory", "Connection aborted", "Connection refused", "Not connected", "Already connected", "Connection closed", "Initialization error (interapplication manager)", "Bad occurrence", "Wait on unbound occurrence handler", "Occurrence queue overflow", "Datalog type conflict", "Unused", "Unrecognized type (interapplication manager)", "Memory corrupt", "Failed to make temporary DLL", "Old CIN version", "Drag socket not found", "Failed to load drop-object", "Failed to register OLE object", "Failed to release OLE object", "Format specifier type mismatch", "Unknown format specifier", "Too few format specifiers", "Too many format specifiers", "Scan failed", "Newer CIN version", "Error converting to variant", "Runtime menu error", "Password tampered", "Variant attribute not found", "Incompatible variant data type", "Event data is not available", "Event Store is not present", "Occurrence is not found", "Event Queue is not created", "Event info is not available", "Refnum passed is NULL", "Error retrieving Class GUID", "Error retrieving CoClass GUID", "Error retrieving TypeLib GUID.", "Bad built application magic bytes.", "Specific driver is different from the specific driver associated with the Logical Name.", "There is no session opened to the class driver.", "Max Error", "MAX - Error with config objects", "MAX - Error loading configuration", "MAX - Group not supported"]
        # "Current State"
        # "Do not delete, rename, or modify this frame.\n(this is used to capture unhandled states and typos)"
        # "Handle mistyped state name (developer tool)"
        n106 = Format Into String(format string="Software Exception: Unhandled State \"%s\"." ("message"), error in=w260, w255) -> (resulting string=w263:string, error out=w262:errorcluster)  [unwired: 1 in]
        n107 = call <vilib>:"Error Cluster From Error Code.vi"("show call chain? (False)"=TRUE, "error in (no error)"=w262, "error message (\"\")"=w263, "error code (0)"=w264) -> ("error out"=w261:errorcluster)  [unwired: 5 in]
        n108 = call <vilib>:"Add State(s) to Queue__jki_lib_state_machine.vi"("State(s) in (\"\")"=w259) -> ("States Out"=w258:string)  [unwired: 14 in]
      }
      frame "Initialize Core Data" {
        # "Do not delete, rename, or modify this frame.\n(this is used to determine panel behavior on exit)"
        # "originally closed?"
        # "exe?"
        # "If panel starts closed or is an EXE, then close it when we exit"
        n109 = property class="VI"() -> ("Front Panel.Open"=w277:bool)  [unwired: 2 in, 2 out]
        n110 = property class="App"() -> ("App.Kind"=w276:T4)  [unwired: 2 in, 2 out]
        n111 = control-ref of="Current VI Reference"() -> (w270:refnum<vi>)
        n112 = Not(x=w277) -> (.not. x?=w274:bool)
        n113 = Equal?(x=w276, y=T4."Run Time System" ("Application:Kind")) -> (x = y?=w273:bool)
        n114 = call-poly <vilib>:"UDP Multicast Open.vi"("time-to-live (1)"=u16 2, "port"="Multicast Local Port") -> ("connection ID"=w268:refnum<k16>)  [unwired: 8 in, 1 out]
        n115 = Or(x=w274, y=w273) -> (x .or. y?=w271:bool)
        n116 = Bundle By Name(cluster=w272, "Core.Current VI Reference"=w270, "Core.Close Panel on Exit?"=w271, "MultiCast connection ID"=w268) -> (w279:T6)
        n117 = property on="SendStop" class="Bool (strict)"("Visible"=FALSE) -> ()  [unwired: 2 in, 2 out]
        n118 = call <vilib>:"Add State(s) to Queue__jki_lib_state_machine.vi"("State(s) in (\"\")"=w281) -> ("States Out"=w280:string)  [unwired: 14 in]
      }
      frame "Error Handler" {
        # "Unhandled Error -- Display it"
        # "Handle any errors here.\nYou can also output any states to clean-up after errors occur"
        # "Clear error"
        n119 = call <vilib>:"General Error Handler.vi"("error in (no error)"=w283) -> ()  [unwired: 10 in, 5 out]
        n120 = call <vilib>:"Add State(s) to Queue__jki_lib_state_machine.vi"("State(s) in Front (\"\")"="/* Post Error States", "State(s) in (\"\")"=w287) -> ("States Out"=w286:string)  [unwired: 13 in]
      }
      frame "Exit" {
        w289 = TRUE
        # "Do not put any code in this frame.\n(No errors that occur here will be handled.)"
        n121 = Unbundle By Name(w293) -> ("MultiCast connection ID"=w292:refnum<k16>)
        n122 = UDP Close(connection ID=w292, 8:w291) -> (error out=w290:errorcluster)  [unwired: 1 out]
        n123 = call <vilib>:"Add State(s) to Queue__jki_lib_state_machine.vi"("State(s) in (\"\")"=w295) -> ("States Out"=w294:string)  [unwired: 14 in]
        n124 = call "Stop_Main_FGV.vi"("Command"=enum16{"set", "get", "init"}."set", "Stop"=w289) -> ()  [unwired: 9 in, 1 out]
      }
      frame "---------- Data ----------" {
        # "Do not put any code in this frame.\n(It is a separator no-op. You can make a copy of this frame to create a new Data frame)"
        n125 = call <vilib>:"Add State(s) to Queue__jki_lib_state_machine.vi"("State(s) in (\"\")"=w299) -> ("States Out"=w298:string)  [unwired: 14 in]
      }
      frame "Data: Initialize" {
        w300 = refnum<k16> refnum  # MultiCast connection ID
        w301 = string[] []  # Devies To Stop
        w303 = T7 {"Current VI Reference"=refnum, "Close Panel on Exit?"=TRUE}  # Core
        w305 = TRUE  # Your Boolean data
        w304 = ""  # Your string data
        # "do not delete - used by framework"
        # "Add new data here."
        # "Data names and types of shift register data are defined by this bundle."
        # "Initialize the shift-register data, here.\n(data names are defined by what you wire into the bundle function)"
        n126 = Bundle("Core"=w303, "Your Boolean data"=w305, "Your string data"=w304, "All connections"=T1[] [], "Devies To Stop"=w301, "MultiCast connection ID"=w300) -> (w307:T6)  [unwired: 1 in]
        n127 = call <vilib>:"Add State(s) to Queue__jki_lib_state_machine.vi"("State(s) in (\"\")"=w309) -> ("States Out"=w308:string)  [unwired: 14 in]
      }
      frame "Data: Cleanup" {
        # "Cleanup any data and references, here.\n(this is called automatically, by the Macro: Exit)"
        n128 = Unbundle By Name(w310) -> ("Core.Current VI Reference"=w313:refnum<vi>)
        n129 = Close Reference(reference=w313, error in (no error)=w312) -> (error out=w311:errorcluster)
        n130 = call <vilib>:"Add State(s) to Queue__jki_lib_state_machine.vi"("State(s) in (\"\")"=w315) -> ("States Out"=w314:string)  [unwired: 14 in]
      }
      frame "---------- UI ----------" {
        # "Do not put any code in this frame.\n(It is a separator no-op. You can make a copy of this frame to create a new UI frame)"
        n131 = call <vilib>:"Add State(s) to Queue__jki_lib_state_machine.vi"("State(s) in (\"\")"=w319) -> ("States Out"=w318:string)  [unwired: 14 in]
      }
      frame "UI: Initialize" {
        # "Initialize the User Interface, here.\n(this is called automatically, by the Macro: Init)"
        n132 = call <vilib>:"Add State(s) to Queue__jki_lib_state_machine.vi"("State(s) in (\"\")"=w323) -> ("States Out"=w322:string)  [unwired: 14 in]
      }
      frame "UI: Cursor Set" {
        # "Argument"
        # "Set and Unset Cursor Busy.\n(Usage: \"UI: Cursor Set >> Busy|Idle\")"
        n133 = case shown="\"Idle\", Default" w324 {
          tunnel: w326 -> [w331 w333]
          tunnel: [w330 w332] -> w325
          frame "Idle", Default {
            n134 = call <vilib>:"Unset Busy.vi"("error in (no error)"=w331) -> ("error out"=w330:errorcluster)  [unwired: 10 in]
          }
          frame "Busy" {
            n135 = call <vilib>:"Set Busy.vi"("error in (no error)"=w333) -> ("error out"=w332:errorcluster)  [unwired: 9 in, 1 out]
          }
        }
        n136 = call <vilib>:"Add State(s) to Queue__jki_lib_state_machine.vi"("State(s) in (\"\")"=w329) -> ("States Out"=w328:string)  [unwired: 14 in]
      }
      frame "UI: Front Panel State" {
        # "Argument"
        # "Set Front Panel Open or Closed\n(Usage: \"UI: Front Panel State >> Open|Close\")"
        n137 = Unbundle By Name(w336) -> ("Core.Current VI Reference"=w335:refnum<vi>)
        n138 = case shown="\"Open\", Default" w334 {
          tunnel: w338 -> [w344 w357]
          tunnel: [w346 w358] -> w337
          tunnel: w335 -> [w345 w355]
          frame "Open", Default {
            n139 = property class="VI"(reference=w345, error in=w344) -> (reference out=w342:refnum<vi>, error out=w343:errorcluster, "Front Panel.Open"=w341:bool)
            n140 = case shown="False" w341 {
              tunnel: [w349 w352] -> w346
              tunnel: w343 -> [w348 w352]
              tunnel: w342 -> [w347 _]
              frame False {
                n141 = invoke class="VI" method="FP.Open"(reference=w347, error in=w348, "Activate"=TRUE, "State"=T5."Standard") -> (error out=w349:errorcluster)  [unwired: 1 in, 4 out]
              }
              frame True {
              }
            }
          }
          frame "Close" {
            n142 = property class="VI"(reference=w355, error in=w357) -> (reference out=w354:refnum<vi>, error out=w356:errorcluster, "Front Panel.Open"=w353:bool)
            n143 = case shown="True" w353 {
              tunnel: [w359 w362] -> w358
              tunnel: w356 -> [w359 w361]
              tunnel: w354 -> [_ w360]
              frame False {
              }
              frame True {
                n144 = invoke class="VI" method="FP.Close"(reference=w360, error in=w361) -> (error out=w362:errorcluster)  [unwired: 1 in, 2 out]
              }
            }
          }
        }
        n145 = call <vilib>:"Add State(s) to Queue__jki_lib_state_machine.vi"("State(s) in (\"\")"=w340) -> ("States Out"=w339:string)  [unwired: 14 in]
      }
      frame "---------- Macro ----------" {
        # "Do not put any code in this frame.\n(It is a separator no-op. You can make a copy of this frame to create a new Macro frame)"
        n146 = call <vilib>:"Add State(s) to Queue__jki_lib_state_machine.vi"("State(s) in (\"\")"=w366) -> ("States Out"=w365:string)  [unwired: 14 in]
      }
      frame "Macro: Initialize" {
        w367 = "Data: Initialize\nInitialize Core Data\nUI: Initialize\nUI: Front Panel State >> Open"  # Data: Initialize Initialize Core Data UI: Initialize UI: Front Panel State >> Open
        # "Initialization Macro\n(This is called once, when the VI starts)"
        n147 = call <vilib>:"Add State(s) to Queue__jki_lib_state_machine.vi"("State(s) in Front (\"\")"=w367, "State(s) in (\"\")"=w371) -> ("States Out"=w370:string)  [unwired: 13 in]
      }
      frame "Macro: Exit" {
        # "Exit Macro\n(This is called once, when the VI exits)"
        n148 = Unbundle By Name(w378) -> ("Core.Close Panel on Exit?"=w373:bool)
        n149 = Select(t="UI: Front Panel State >> Close", s=w373, f="") -> (s? t:f=w376:string)
        n150 = call <vilib>:"Add State(s) to Queue__jki_lib_state_machine.vi"("State(s) in (\"\")"=w376, "State(s) at Back (\"\")"="Data: Cleanup\nExit") -> ("States Out"=w372:string)  [unwired: 13 in]
        n151 = call <vilib>:"Add State(s) to Queue__jki_lib_state_machine.vi"("State(s) in Front (\"\")"=w372, "State(s) in (\"\")"=w381) -> ("States Out"=w380:string)  [unwired: 13 in]
      }
      frame "---------- Main ----------" {
        # "Template Separator\n(You can make a copy of, or modify, this frame)"
        n152 = call <vilib>:"Add State(s) to Queue__jki_lib_state_machine.vi"("State(s) in (\"\")"=w385) -> ("States Out"=w384:string)  [unwired: 14 in]
      }
      frame "Main: Send Stop Command" {
        # "Your code here.\n(You can make a copy of, or modify, this frame)"
        n153 = Unbundle By Name(w388) -> ("All connections"=w386:T1[], "Devies To Stop"=w387:string[])
        n154 = for {
          tunnel: w387 -> [w392] mode=indexing
          tunnel: w386 -> [w393]
          n155 = for {
            tunnel: w393 -> [w394] mode=indexing
            tunnel: w392 -> [w396]
            n156 = Unbundle By Name(w394) -> ("Name"=w397:string)
            n157 = Equal?(x=w397, y=w396) -> (x = y?=w395:bool)
            n158 = case shown="True" w395 {
              tunnel: w394 -> [_ w405]
              frame False {
              }
              frame True {
                w401 = ">>" ("string")
                n159 = Unbundle By Name(w405) -> ("connection ID"=w404:refnum<k5>, "Name"=w403:string, "IP address"=w402:string)
                n160 = Concatenate Strings(w403, w401, w402, w401, "Stop" ("string")) -> (w399:string)
                n161 = String Length(string=w399) -> (length=w407:i32)
                n162 = Type Cast(type=w399, x=w407) -> (*(type *) &x=w406:string)
                n163 = TCP Write(connection ID=w404, data in=w406) -> (connection ID out=w408:refnum<k5>, error out=w409:errorcluster)  [unwired: 2 in, 1 out]
                n164 = TCP Write(connection ID=w408, data in=w399, error in (no error)=w409) -> (error out=w398:errorcluster)  [unwired: 1 in, 2 out]
                n165 = call <vilib>:"Clear Errors.vi"("error in (no error)"=w398) -> ()  [unwired: 5 in, 2 out]
              }
            }
          }
        }
        n166 = call <vilib>:"Add State(s) to Queue__jki_lib_state_machine.vi"("State(s) in (\"\")"=w391) -> ("States Out"=w390:string)  [unwired: 14 in]
      }
      frame "Main: ClearList" {
        # "Your code here.\n(You can make a copy of, or modify, this frame)"
        n167 = call "Connection Alive FGV A.vi"("command"=Command."return all connections") -> ("all connections"=w412:refnum<k5>[], "Names"=w411:string[])  [unwired: 7 in, 6 out]
        n168 = for {
          tunnel: w412 -> [w419] mode=indexing
          tunnel: w411 -> [_] mode=indexing
          n169 = call "Connection Alive FGV A.vi"("command"=Command."remove connection", "connection ID"=w419) -> ()  [unwired: 6 in, 8 out]
        }
        n170 = call <vilib>:"Add State(s) to Queue__jki_lib_state_machine.vi"("State(s) in Front (\"\")"="Main: Refresh Connections" ("State(s) in Front (\"\")"), "State(s) in (\"\")"=w417) -> ("States Out"=w416:string)  [unwired: 13 in]
      }
      frame "Main: Refresh Connections" {
        # "Your code here.\n(You can make a copy of, or modify, this frame)"
        n171 = call "Connection Alive FGV A.vi"("command"=Command."return all connections") -> ("All connections"=w428:T1[], "Names"=w427:string[], "IP Addresses"=w426:string[])  [unwired: 7 in, 5 out]
        "All connections" <- w428
        n172 = Build Array(w427, w426) -> (w425:string[][])
        n173 = Transpose 2D Array(2D array=w425) -> (transposed array=w424:string[][])
        n174 = property on="Listbox" class="LstBox (strict)"("Item Names"=w427) -> ()  [unwired: 2 in, 2 out]
        n175 = property on="Multicolumn Listbox" class="MCListbox (strict)"("ItemNames"=w424, "NumCols"=u32 2 ("Number of Columns"), "ColHdrString"=string[] ["Name", "Location"] ("Column Header Strings[]")) -> ()  [unwired: 2 in, 2 out]
        n176 = Bundle By Name(cluster=w421, "All connections"=w428) -> (w420:T6)
        n177 = call <vilib>:"Add State(s) to Queue__jki_lib_state_machine.vi"("State(s) in (\"\")"=w432) -> ("States Out"=w431:string)  [unwired: 14 in]
      }
    }
  }
  n178 = call <vilib>:"Clear Errors.vi"("error in (no error)"=w12) -> ("error out"=w10:errorcluster)  [unwired: 5 in, 1 out]
  n179 = TCP Close Connection(connection ID=w13, error in (no error)=w10) -> (error out=w2:errorcluster)  [unwired: 2 out]
  n180 = flat-sequence {
    tunnel: w2 -> [_]
    frame #0 {
      n181 = local write "Exit"(FALSE ("OK")) -> ()
    }
  }
